vi "Dashboard Main.vi"() -> ()   [LabVIEW 2018]
uses:
  <vilib>/Utility/miscctls.llb/LVRowAndColumnTypeDef.ctl
  <vilib>/event_ctls.llb/eventvkey.ctl
  <vilib>/Rock Robotics/Network Tables/NT Read Numeric Array.vi
  <vilib>/Rock Robotics/Network Tables/NT Write Boolean.vi
  <vilib>/Rock Robotics/WPI/Dashboard/WPI_DashboardLogging Global.vi
  <vilib>/Rock Robotics/Network Tables/NT Write Numeric Array.vi
  <vilib>/Rock Robotics/Network Tables/NT Read Boolean Array.vi
panel:
  out "Time":dbl
  out "Boolean Array":bool[](array[boolean])
  in  "Key Binds":u16[](array[ring]) items=["No Function", "Gear Shift", "Direction Toggle", "Cube Up", "Cube Down", "LRamp Deploy", "RRamp Deploy", "LRamp Raise", "RRamp Raise"]
  in  "Turning Multiplier":dbl=1.0 format="%#_13g"
  in  "Control System":T1(ring)
  out "error out 2":errorcluster
  out "Profile Name":string="Profile1"
  in  "Load":bool
  in  "Save":bool
  in  "High Gear Turning Multiplier":dbl=0.65 format="%#_13g"
  in  "Turning Deadzone":dbl=0.4 format="%#_13g"
  in  "Foreward Deadzone":dbl=1.0 format="%#_13g"
  in  "Max Speed":dbl=1.0 format="%#_13g"
  in  "Autoshift":bool=TRUE
  in  "Direction Toggle":bool=TRUE
  in  "High Gear":bool=TRUE
  in  "Camera Settings Right":T2={"Frame Rate"=30, "Compression"=30, "Size"=1, "DB Camera Config"=FALSE} {"Frame Rate" scale=1.0..30.0; "Compression" scale=100.0..-1.0; "Size" items=["640x480", "320x240", "160x120"]}
  in  "Camera Name Right":string(combo)="No Camera Selection"
  out "Camera Perf":string
  in  "Camera Settings":T2={"Frame Rate"=30, "Compression"=30, "Size"=1, "DB Camera Config"=FALSE} {"Frame Rate" scale=1.0..30.0; "Compression" scale=100.0..-1.0; "Size" items=["640x480", "320x240", "160x120"]}
  in  "TCP":refnum<k5>
  in  "Rec Mode":enum32{"Stop", "Record", "Playback"}(radio)
  out "Robot IP":string
  out "Image Message":string="Timeout in Camera Communications"
  in  "Dashboard Tab":T3(tab)
  in  "Select Auto":string(combo)="Select Autonomous ..."
  out "NT Connection":bool
  out "MotorChart R":cluster{"Numeric":dbl, "Numeric":dbl}(graph)
  out "MotorChart L":cluster{"Numeric":dbl, "Numeric":dbl}(graph)
  out "MotorSliders R":cluster{"MotorSlide1":dbl, "MotorSlide2":dbl} {"MotorSlide2" scale=-1.0..1.0 scale format="%#_2e"; "MotorSlide1" scale=-1.0..1.0 scale format="%#_2e"}
  out "MotorSliders L":cluster{"MotorSlide1":dbl, "MotorSlide2":dbl} {"MotorSlide2" scale=-1.0..1.0 scale format="%#_2e"; "MotorSlide1" scale=-1.0..1.0 scale format="%#_2e"}
  out "Gyro":dbl(knob) scale=0.0..360.0
  out "JS1 Z":dbl(slide) scale=-1.0..1.0 scale format="%#_2e"
  out "JS1 Graph":cluster{"X":dbl, "Y":dbl}[](graph)
  out "JS1 Buttons":T4
  out "JS2 Z":dbl(slide) scale=-1.0..1.0 scale format="%#_2e"
  out "JS2 Graph":cluster{"X":dbl, "Y":dbl}[](graph)
  out "JS2 Buttons":T4
  out "Mode":T5(ring)=enum."Auto Disabled"
  out "Right Camera Perf":cluster{"Bandwidth (Mbps)":dbl, "FPS":dbl}
  out "Camera Image Right":T6(plugin-control)
  in  "DB/String 9":string
  in  "DB/String 8":string
  in  "DB/String 7":string
  in  "DB/String 6":string
  in  "DB/String 5":string
  in  "DB/String 4":string
  in  "DB/String 3":string
  in  "DB/String 2":string
  in  "DB/String 1":string
  in  "DB/String 0":string
  in  "DB/Slider 0":dbl(slide) scale=0.0..5.0
  in  "DB/Slider 1":dbl(slide) scale=0.0..5.0
  in  "DB/Slider 2":dbl(slide) scale=0.0..5.0
  in  "DB/Slider 3":dbl(slide) scale=0.0..5.0
  out "DB/LED 3":bool
  out "DB/LED 2":bool
  out "DB/LED 1":bool
  out "DB/LED 0":bool
  in  "DB/Button 3":bool
  in  "DB/Button 2":bool
  in  "DB/Button 1":bool
  in  "DB/Button 0":bool caption="New Name"
  in  "Toggle Interpolation":bool
  out "XY Graph":cluster{dbl[], dbl[]}(graph)
  in  "Add Cursor":bool
  in  "Interpolation Method":i32(ring)=1 items=["nearest", "linear", "spline", "cubic Hermite", "Lagrange"]
  in  "Graph Points":i32
  in  "Remove Cursor":bool
  in  "Test Slider":dbl(slide) scale=0.0..100.0 scale format="%#_3g"
  in  "On/Off":bool caption="Solenoid"
  in  "Test Name":u16(ring) items=["Select the test to run..."]
  in  "Test Tree":string(tree)
  in  "Motor":cluster{"Value":dbl, "Enable":bool} {"Value" scale=-1.0..1.0 scale format="%#_3g"}
  out "Progress":T7 {"Test Progress" scale=0.0..100.0}
  in  "Rev/Fwd":cluster{"Forward":bool, "Reverse":bool}
  in  "Test Ring":u16(ring) items=["Monochrome", "Color"]
  out "Cmd Status":string
  in  "Execute Command":bool
  in  "Command Params":string[][](table)
  in  "Command Selection":i32(listbox)
  in  "CheckList":i32(listbox)
  out "Tree":string(tree)
  out "Camera Image":T6(plugin-control)
  out "Background":bool
  in  "Camera Name":string(combo)="No Camera Selection"
  # "HW"
  # "HW"
  # "Raw Joystick"
  # "Interpolated Joystick"
  # "Drive Motors"
  # "Front"
  # "Right"
  # "Left"
  # "Back"
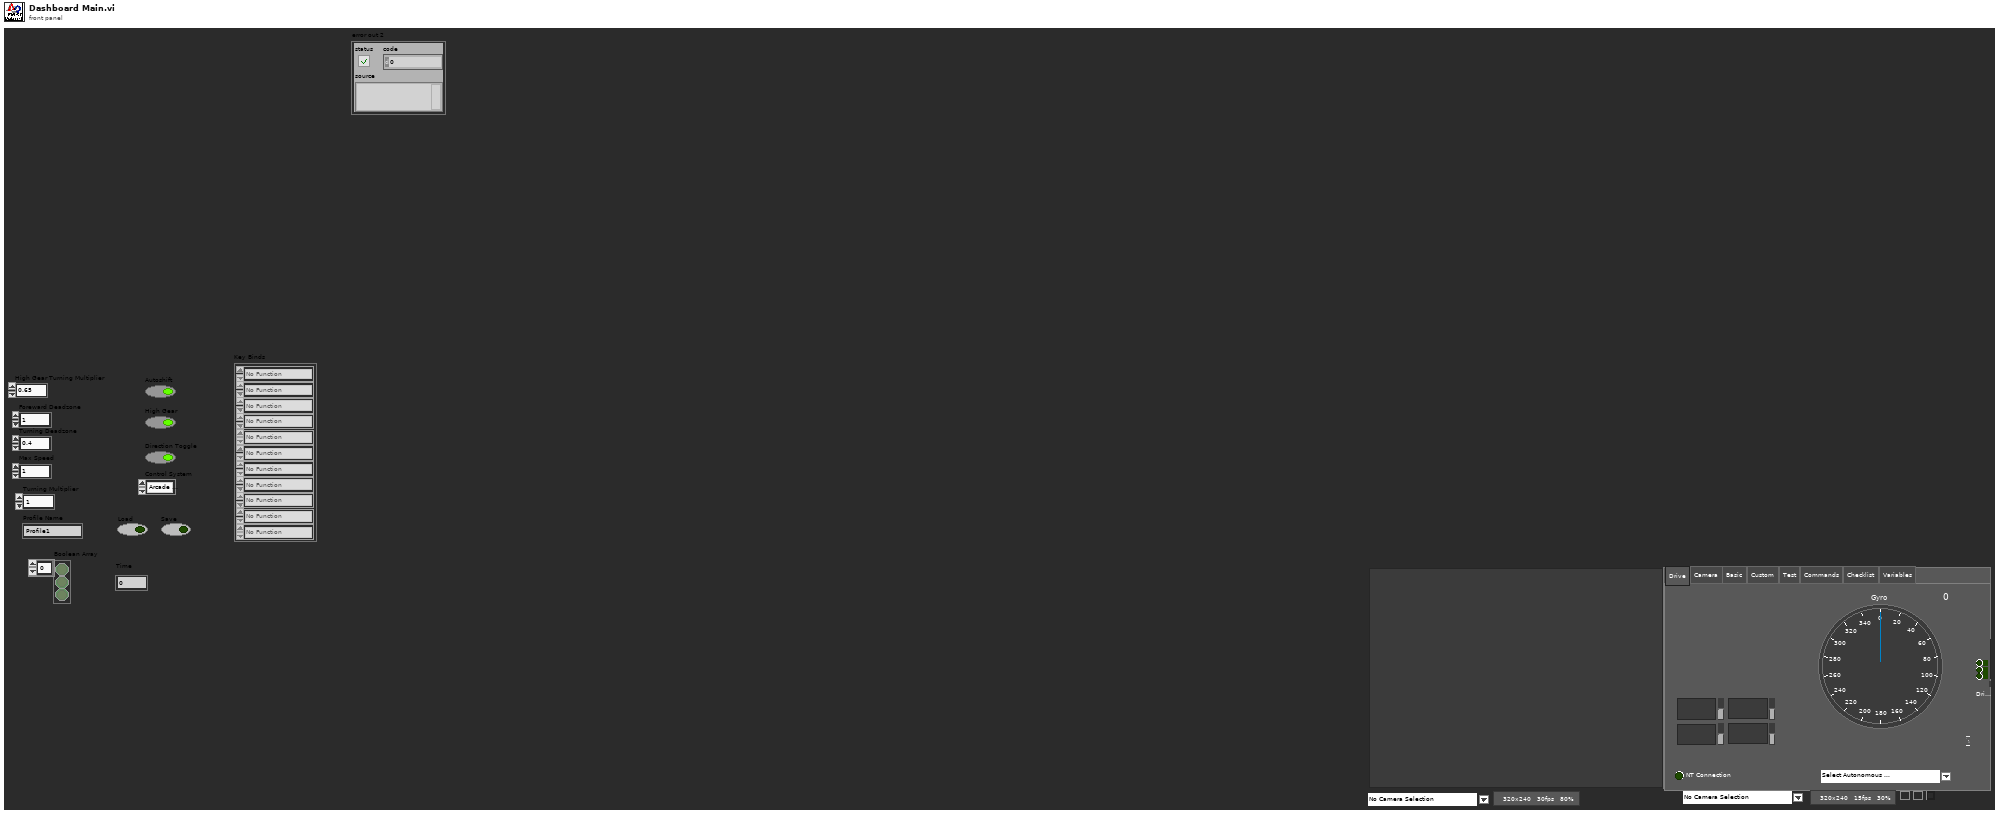
[diagram p1: front panel]
types:
  T1 = enum16{"Arcade Drive", "Two Part Arcade Drive", "Tank"}
  T2 = cluster{"Frame Rate":i32, "Compression":i32, "Size":u16, "DB Camera Config":bool}
  T3 = enum32{"Drive", "Camera", "Basic", "Custom", "Test", "Commands", "Checklist", "Variables"}
  T4 = cluster{bool, bool, bool, bool, bool, bool, bool, bool, bool, bool, bool, bool}
  T5 = enum8{"Tele-Op Disabled", "Tele-Op Enabled", "Auto Disabled", "Auto Enabled", "Test Disabled", "Test Enabled", "Disconnected", "No Code", "E-Stop"}
  T6 = typedef "IMAQ Image.ctl" = refnum<image>
  T7 = cluster{"Test Progress":u8, "Test Progress Text":string}
  T8 = cluster{"Save Path":path, "Interval (s)":dbl, "Keep":i32}
  T9 = typedef "Image Type" = u32
  T10 = cluster{"IDs":cluster{"RPC field ID":u16, "Unique ID":u16}, "String":string}
  T11 = cluster{"High Gear Turning Multiplier":refnum<vi>, "Turning Deadzone":refnum<vi>, "Foreward Deadzone":refnum<vi>, "Max Speed":refnum<vi>, "Autoshift":refnum<vi>, "High Gear":refnum<vi>, "Direction Toggle":refnum<vi>, "Control System":refnum<vi>, "Turning Multiplier":refnum<vi>, "Profile Name":refnum<vi>, "Key Binds":refnum<vi>}
  T12 = cluster{"Error Strings":string, "Disable Counts":cluster{u16, u16}, "Rail Faults":cluster{u16, u16, u16}, "Robot IP":string, "DB Mode":u8, "Event Info":cluster{"Name":string, "Type":u8, "Number":u16, "Replay":u8}}
  T13 = cluster{"Storage":cluster{"Disk Free":u64, "RAM Block":u32, "RAM free":u32}, "CPU Utilization":cluster{"CPU % ISR":sgl, "CPU % Time Crit":sgl, "CPU % Timed Str":sgl, "CPU % High":sgl, "CPU % Above":sgl, "CPU % Normal":sgl, "CPU % Low":sgl}, "CAN":cluster{"% Bus Utilization":sgl, "Bus Off Cnt":u32, "TX_FIFO Full Cnt":u32, "Receive Error Cnt":u8, "Transmit Error Cnt":u8}, "HID":cluster{"HID Outputs":u32, "Rumble Low":u16, "Rumble High":u16}[]}
  T14 = cluster{"Status bits":cluster{"Test Mode":bool, "Autonomous":bool, "Enabled":bool, "Code Start":bool, "Brownout":bool, "Reserved 2":bool, "Reserved 3":bool, "E-Stop":bool}, "Code Trace":cluster{"Disabled":bool, "TeleOp":bool, "Auto":bool, "Test":bool}, "Controller Type":enum16{"unknown", "cRIO", "roboRio"}, "Code?":enum16{"unknown", "noCode", "code"}, "Battery V":dbl}
  T15 = cluster{"Control Bits":cluster{"TestMode":bool, "Autonomous":bool, "Enabled":bool, "FMS Present":bool, bool, bool, bool, "E-Stop":bool}, "Team Station ":u8, "Countdown":sgl, "Joystick Values":cluster{"Axes":dbl[], "Buttons":bool[], "POVs":i16[]}[]}
  T16 = cluster{"Axes":dbl[], "Buttons":bool[], "POVs":i16[]}[]
  T17 = cluster{"Axes":dbl[], "Buttons":bool[], "POVs":i16[]}
  T18 = cluster{"Buttons[0]":bool, "Buttons[1]":bool, "Buttons[2]":bool, "Buttons[3]":bool, "Buttons[4]":bool, "Buttons[5]":bool, "Buttons[6]":bool, "Buttons[7]":bool, "Buttons[8]":bool, "Buttons[9]":bool, "Buttons[10]":bool, "Buttons[11]":bool}
  T19 = cluster{"Camera Image":refnum<vi>, "Dashboard Tab":refnum<vi>, "Background":refnum<vi>, "Rec Mode":refnum<vi>, "Test Slider":refnum<vi>, "On/Off ":refnum<vi>, "Test Ring":refnum<vi>, "Rev/Fwd":refnum<vi>, "Test Name":refnum<vi>, "Motor":refnum<vi>, "Progress":refnum<vi>, "CheckList":refnum<vi>, "Tree":refnum<vi>, "Test Tree":refnum<vi>, "Command Params":refnum<vi>, "Command Selection":refnum<vi>, "Execute Command":refnum<vi>, "Cmd Status":refnum<vi>, "Camera Settings":refnum<vi>, "Camera Name":refnum<vi>, "Camera Perf":refnum<vi>, "Camera Settings Right":refnum<vi>, "Camera Name Right":refnum<vi>, "Camera Image Right":refnum<vi>}
  T20 = cluster{"Global Rectangle":i32[], "Contours":cluster{"Contour Type":u32, "ROI Type":u32, "Points":i32[]}[]}
  T21 = cluster{"Camera Name Right":string, string, "Saved DB Images Info":cluster{"Save Path":path, "Interval (s)":dbl, "Keep":i32}}
  T22 = cluster{"Camera Name":string, string, "Saved DB Images Info":cluster{"Save Path":path, "Interval (s)":dbl, "Keep":i32}}
  T23 = cluster{"Operation":enum16{"Update", "Clear"}, "Color Box":u32}[]
  T24 = typedef "eventvkey.ctl" = enum16{"ASCII", "Enter", "Return", "Shift", "Ctrl", "Alt", "Cmd", "Opt", "Caps", "NumLock", "Clear", "Break", "Up", "Down", "Left", "Right", "Insert", "Delete", "Home", "End", "PageUp", "PageDown", "Escape", "Help", "Pause", "ScrollLock", "F1", "F2", "F3", "F4", "F5", "F6", "F7", "F8", "F9", "F10", "F11", "F12", "F13", "F14", "F15", "F16", "F17", "F18", "F19", "F20", "F21", "F22", "F23", "F24", "Play", "VolumeUp", "VolumeDown", "Mute", "Two Byte Char"}
  T25 = cluster{"Image Size":bool, "Image Type":bool, "Pixel Value":bool, "ROI Information":bool, "Zoom Factor":bool}
  T26 = cluster{"Operation":enum16{"Update", "Clear"}, "Color Box":u32}
  T27 = typedef "LVRowAndColumnTypeDef.ctl" = cluster{"Row":i32, "Column":i32}
  T28 = cluster{"Shift":bool, "Ctrl":bool, "Alt":bool, "Cmd":bool, "Opt":bool}
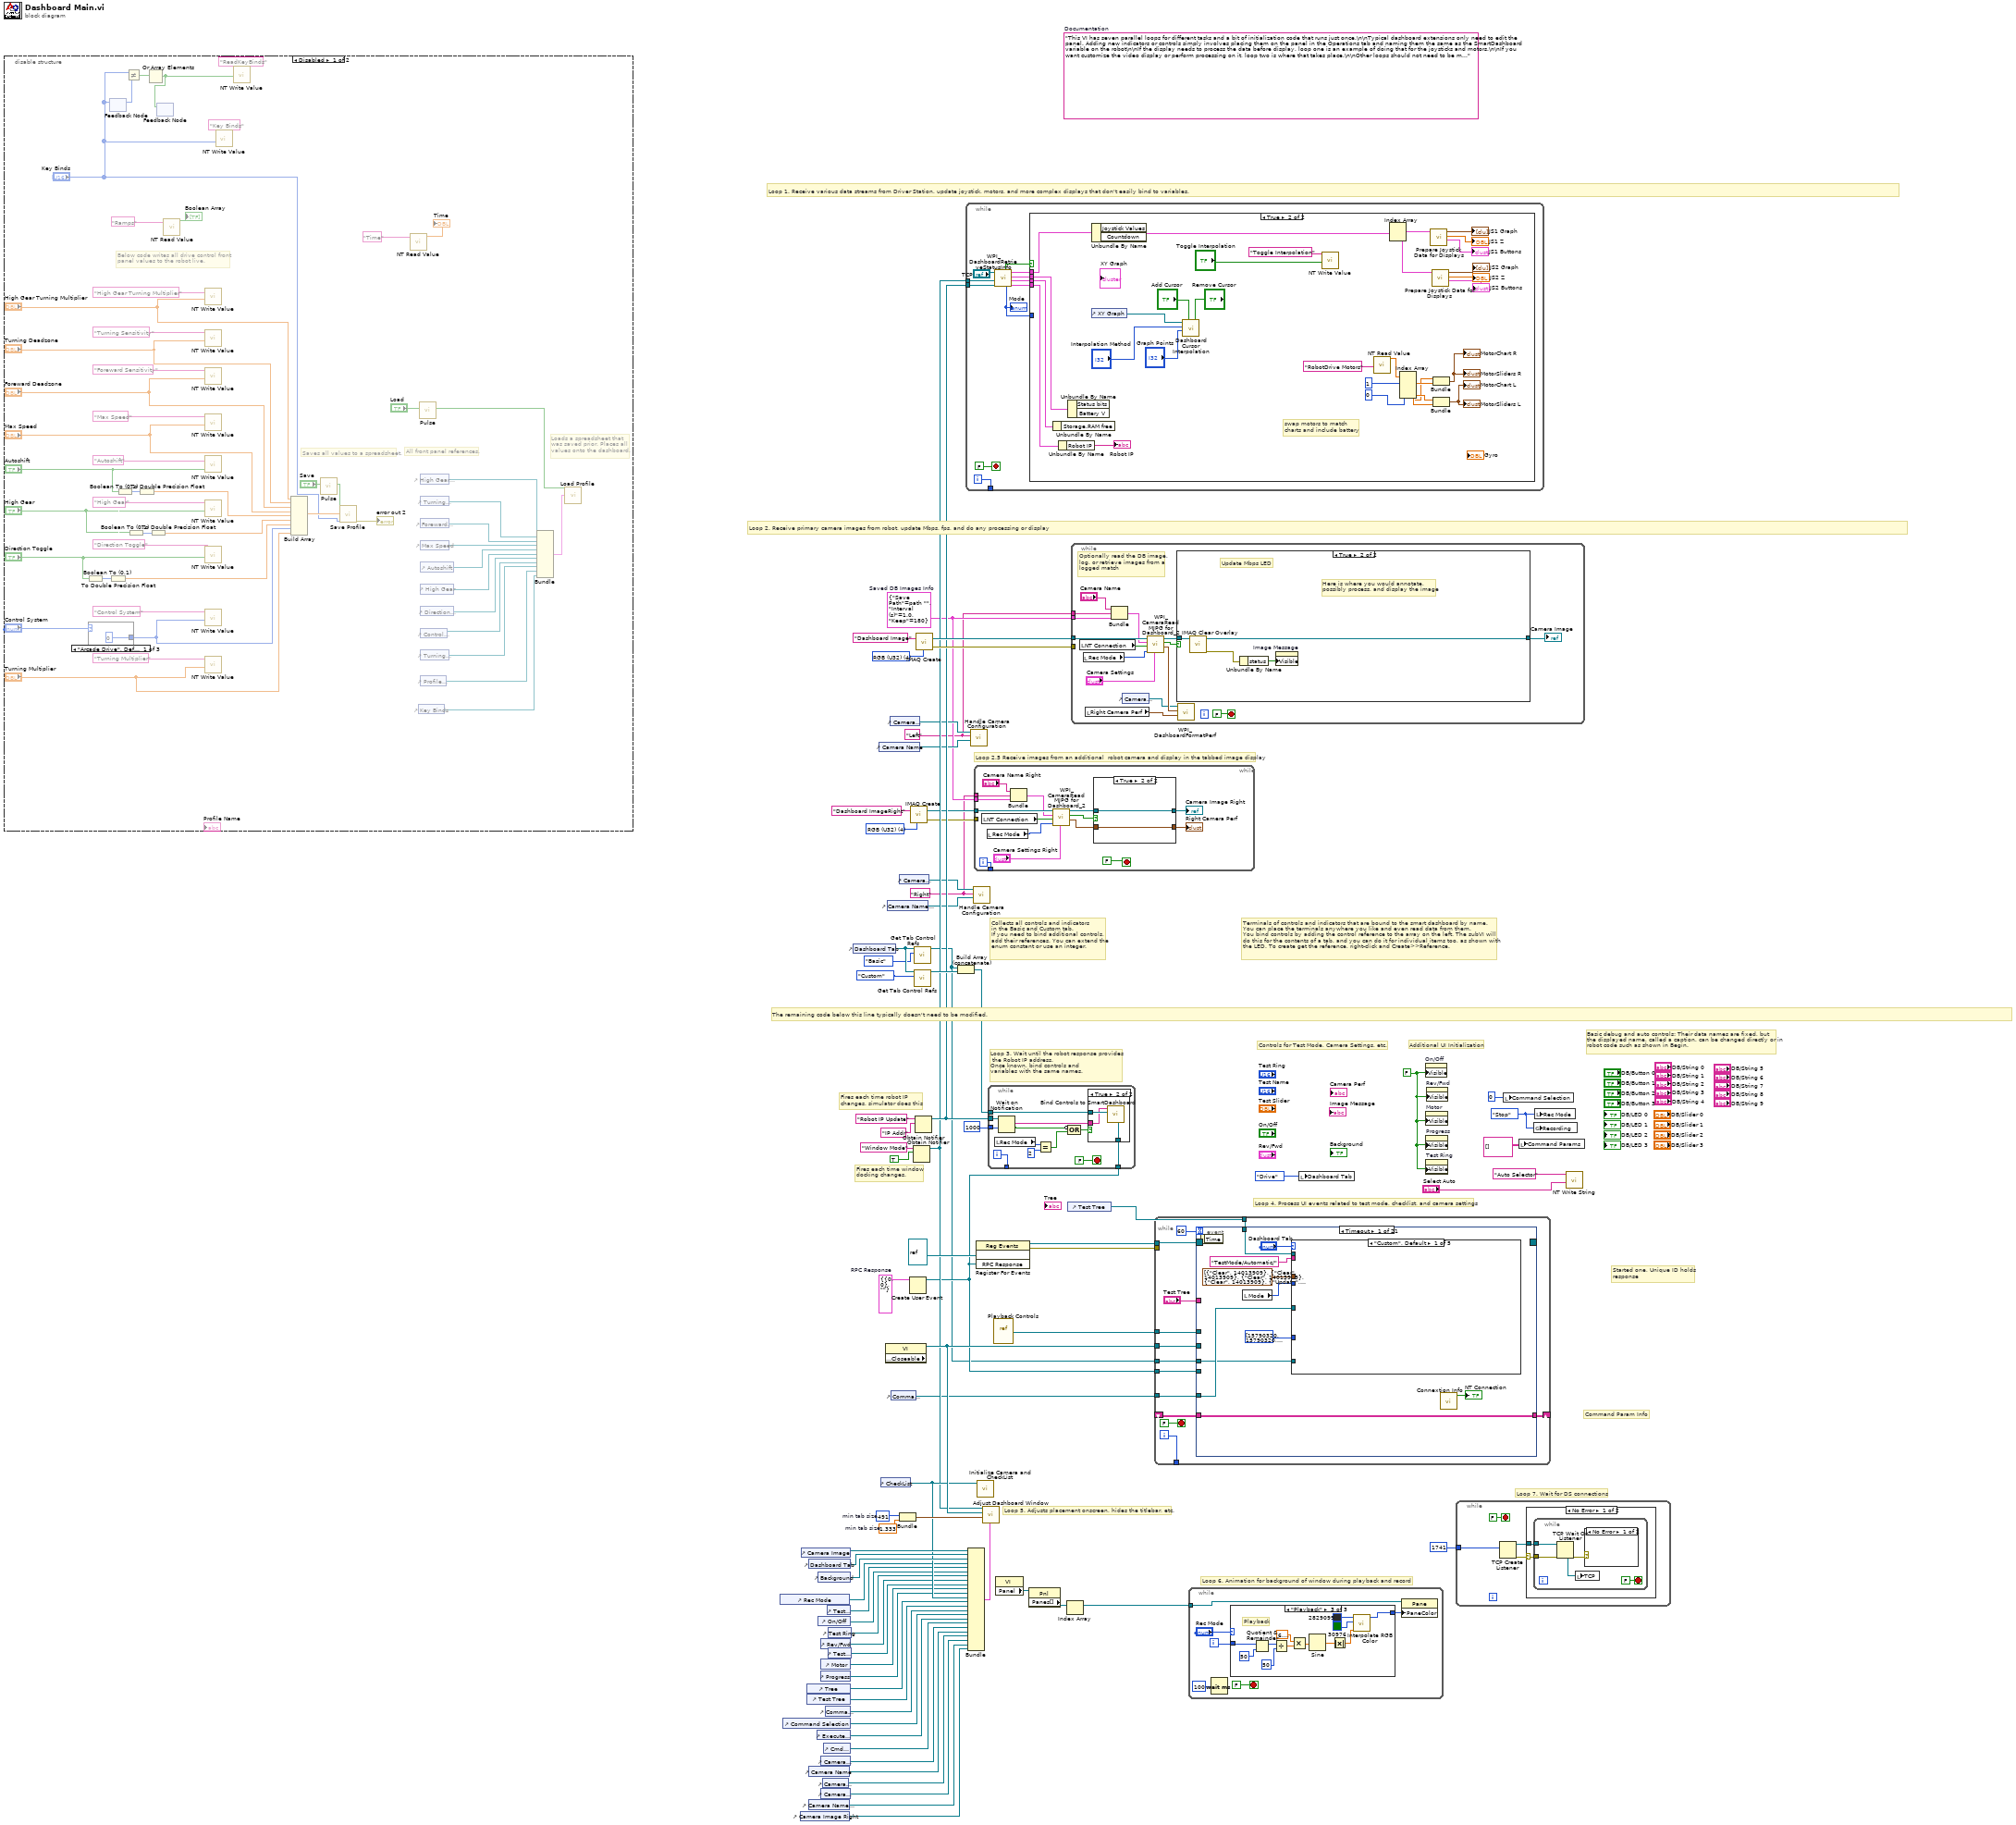
[diagram p0: block diagram]
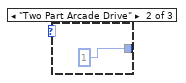
[diagram p2: hidden frame]
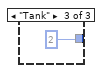
[diagram p3: hidden frame]
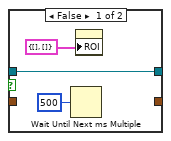
[diagram p5: hidden frame]
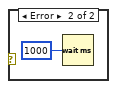
[diagram p6: hidden frame]
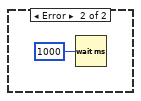
[diagram p7: hidden frame]
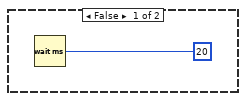
[diagram p8: hidden frame]
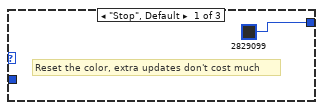
[diagram p9: hidden frame]
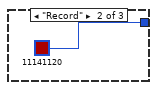
[diagram p10: hidden frame]
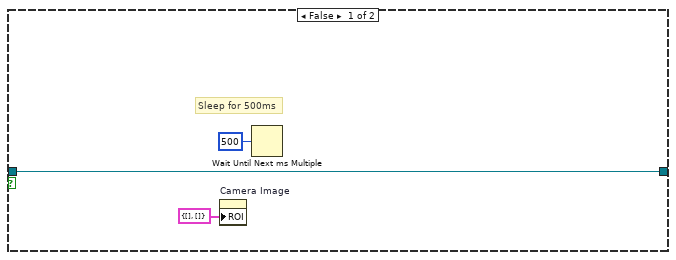
[diagram p12: hidden frame]
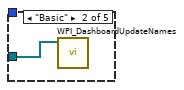
[diagram p13: hidden frame]
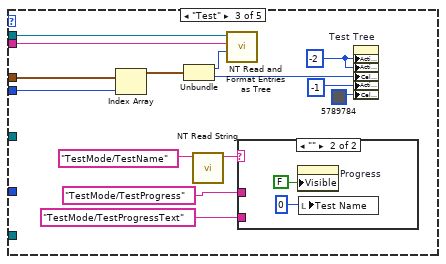
[diagram p14: hidden frame]
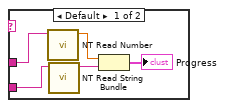
[diagram p15: hidden frame]
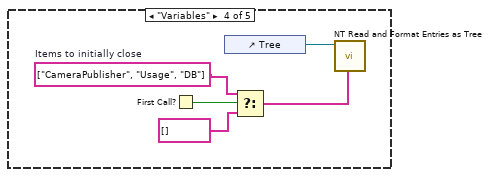
[diagram p16: hidden frame]
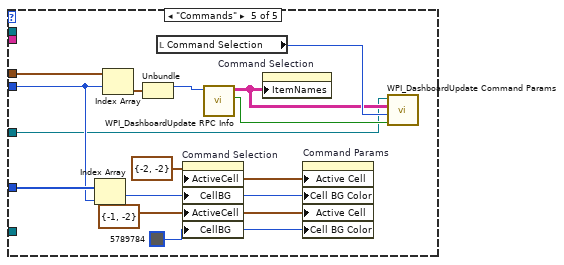
[diagram p17: hidden frame]
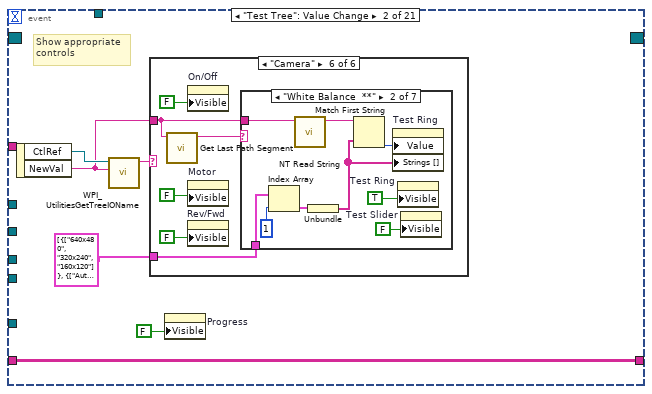
[diagram p18: hidden frame]
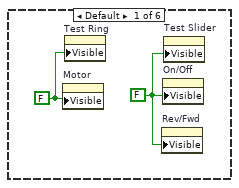
[diagram p19: hidden frame]
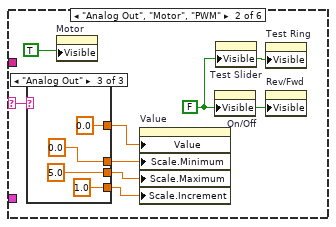
[diagram p20: hidden frame]
diagram:
  w3 = T8 {"Save Path"=path "", "Interval (s)"=1.0, "Keep"=180}  # Saved DB Images Info
  w2 = "Right"
  w1 = "Left"
  w13 = T9 4 items=["Grayscale (U8)", "Grayscale (I16)", "Grayscale (SGL)", "Complex (CSG)", "RGB (U32)", "HSL (U32)", "RGB (U64)"] ("Image Type")
  w29 = T10 {"IDs"={"RPC field ID"=0, "Unique ID"=0}, "String"=""}  # RPC Response
  w52 = 491  # min tab size
  w51 = 1.333  # min tab size
  w59 = enum32{"Stop", "Record", "Playback"}."Stop" ("Rec Mode")
  w36 = FALSE ("Visible")
  (unwired) "This VI has seven parallel loops for different tasks and a bit of initialization code that runs just once.\n\nTypical dashboard extensions only need to edit the panel. Adding new indicators or controls simply involves placing them on the panel in the Operations tab and naming them the same as the SmartDashboard variable on the robot\n\nIf the display needs to process the data before display, loop one is an example of doing that for the joysticks and motors.\n\nIf you want customize the video display or perform processing on it, loop two is where that takes place.\n\nOther loops should not need to be modified. They are pretty standard, and document the task they perform."  # Documentation
  w76 = T9 4 items=["Grayscale (U8)", "Grayscale (I16)", "Grayscale (SGL)", "Complex (CSG)", "RGB (U32)", "HSL (U32)", "RGB (U64)"] ("Image Type")
  # "Loop 2.5 Receive images from an additional  robot camera and display in the tabbed image display"
  # "Command Param Info"
  # "Started one, Unique ID holds\nresponse"
  # "Loop 7. Wait for DS connections"
  # "Basic debug and auto controls: Their data names are fixed, but\nthe displayed name, called a caption, can be changed directly or in\nrobot code such as shown in Begin."
  # "Controls for Test Mode, Camera Settings, etc."
  # "Additional UI Initialization"
  # "Loop 6. Animation for background of window during playback and record"
  # "Fires each time robot IP\nchanges, simulator does this"
  # "Fires each time window\ndocking changes."
  # "Collects all controls and indicators\nin the Basic and Custom tab.\nIf you need to bind additional controls,\nadd their references. You can extend the\nenum constant or use an integer."
  # "The remaining code below this line typically doesn't need to be modified."
  # "Loop 4. Process UI events related to test mode, checklist, and camera settings"
  # "Terminals of controls and indicators that are bound to the smart dashboard by name.\nYou can place the terminals anywhere you like and even read data from them.\nYou bind controls by adding the control reference to the array on the left. The subVI will\ndo this for the contents of a tab, and you can do it for individual items too, as shown with\nthe LED. To create get the reference, right-click and Create>>Reference."
  # "Loop 3. Wait until the robot response provides\n the Robot IP address.\nOnce known, bind controls and\nvariables with the same names."
  # "Loop 5. Adjusts placement onscreen, hides the titlebar, etc."
  # "Loop 1. Receive various data streams from Driver Station, update joystick, motors, and more complex displays that don't easily bind to variables."
  # "Loop 2. Receive primary camera images from robot, update Mbps, fps, and do any processing or display"
  n1 = disable-structure shown="Disabled" {
    frame Disabled {
      # "Loads a spreadsheet that\nwas saved prior. Places all\nvalues onto the dashboard."
      # "All front panel references."
      # "Saves all values to a spreadsheet."
      # "Below code writes all drive control front\npanel values to the robot live."
      n2 = Boolean To (0,1)(Boolean="Direction Toggle") -> (0, 1=w112:i16)
      n3 = case shown="\"Arcade Drive\", Default" "Control System" {
        tunnel: [0 1 2] -> w89
        frame "Arcade Drive", Default {
        }
        frame "Two Part Arcade Drive" {
        }
        frame "Tank" {
        }
      }
      n4 = feedback #1() -> (w88:u16[])  [unwired: 1 in]
      n5 = feedback-in #1("Key Binds") -> ()
      n6 = To Double Precision Float(number=w112) -> (double precision float=w113:dbl)
      n7 = Boolean To (0,1)(Boolean="Autoshift") -> (0, 1=w108:i16)
      n8 = Not Equal?(x="Key Binds", y=w88) -> (x != y?=w87:bool[])
      n9 = Boolean To (0,1)(Boolean="High Gear") -> (0, 1=w110:i16)
      n10 = To Double Precision Float(number=w108) -> (double precision float=w109:dbl)
      n11 = Or Array Elements(Boolean array=w87) -> (logical OR=w85:bool)
      n12 = To Double Precision Float(number=w110) -> (double precision float=w111:dbl)
      n13 = feedback #2() -> ()  [unwired: 2 in]
      n14 = feedback-in #2(w85) -> ()
      n15 = call-poly <vilib>:"NT Read Value.vi"("Name"="Ramps") -> ("Boolean Array"=→"Boolean Array":bool[])  [unwired: 9 in, 1 out]
      n16 = call-poly <vilib>:"NT Write Value.vi"("Numeric"="High Gear Turning Multiplier", "Name"="High Gear Turning Multiplier") -> ()  [unwired: 9 in, 1 out]
      n17 = call-poly <vilib>:"NT Write Value.vi"("Numeric"="Turning Deadzone", "Name"="Turning Sensitivity") -> ()  [unwired: 9 in, 1 out]
      n18 = call-poly <vilib>:"NT Write Value.vi"("Numeric"="Foreward Deadzone", "Name"="Foreward Sensitivity") -> ()  [unwired: 9 in, 1 out]
      n19 = call-poly <vilib>:"NT Write Value.vi"("Numeric"="Max Speed", "Name"="Max Speed") -> ()  [unwired: 9 in, 1 out]
      n20 = call-poly <vilib>:"NT Write Value.vi"("Boolean"="Autoshift", "Name"="Autoshift") -> ()  [unwired: 9 in, 1 out]
      n21 = call-poly <vilib>:"NT Write Value.vi"("Boolean"="High Gear", "Name"="High Gear") -> ()  [unwired: 9 in, 1 out]
      n22 = call-poly <vilib>:"NT Write Value.vi"("Boolean"="Direction Toggle", "Name"="Direction Toggle") -> ()  [unwired: 9 in, 1 out]
      n23 = call-poly <vilib>:"NT Write Value.vi"("Numeric"=w89, "Name"="Control System") -> ()  [unwired: 9 in, 1 out]
      n24 = call-poly <vilib>:"NT Write Value.vi"("Numeric"="Turning Multiplier", "Name"="Turning Multiplier") -> ()  [unwired: 9 in, 1 out]
      n25 = call-poly <vilib>:"NT Write Value.vi"("Numeric Array"="Key Binds", "Name"="Key Binds") -> ()  [unwired: 9 in, 1 out]
      n26 = call-poly <vilib>:"NT Write Value.vi"("Boolean"=w85, "Name"="ReadKeyBinds") -> ()  [unwired: 9 in, 1 out]
      n27 = Build Array("High Gear Turning Multiplier", "Turning Deadzone", "Foreward Deadzone", "Max Speed", w109, w111, w113, w89, "Turning Multiplier") -> (w115:dbl[])
      n28 = call "Pulse.vi"("Input"="Save") -> ("Output"=w107:bool)  [unwired: 10 in]
      n29 = call "Save Profile.vi"("Key Binds"="Key Binds", "Driver Pref"=w115, "Output"=w107) -> ("error out"=→"error out 2":errorcluster)  [unwired: 8 in]
      n30 = call-poly <vilib>:"NT Read Value.vi"("Name"="Time") -> ("Numeric"=→"Time":dbl)  [unwired: 9 in, 1 out]
      n31 = control-ref of="Key Binds"() -> (w83:refnum<vi>)
      n32 = call "Pulse.vi"("Input"="Load") -> ("Output"=w104:bool)  [unwired: 10 in]
      n33 = control-ref of="Profile Name"() -> (w92:refnum<vi>)
      n34 = control-ref of="High Gear Turning Multiplier"() -> (w103:refnum<vi>)
      n35 = control-ref of="Turning Deadzone"() -> (w102:refnum<vi>)
      n36 = control-ref of="Foreward Deadzone"() -> (w101:refnum<vi>)
      n37 = control-ref of="Max Speed"() -> (w100:refnum<vi>)
      n38 = control-ref of="Autoshift"() -> (w99:refnum<vi>)
      n39 = control-ref of="High Gear"() -> (w98:refnum<vi>)
      n40 = control-ref of="Direction Toggle"() -> (w97:refnum<vi>)
      n41 = control-ref of="Control System"() -> (w95:refnum<vi>)
      n42 = control-ref of="Turning Multiplier"() -> (w91:refnum<vi>)
      n43 = Bundle("High Gear Turning Multiplier"=w103, "Turning Deadzone"=w102, "Foreward Deadzone"=w101, "Max Speed"=w100, "Autoshift"=w99, "High Gear"=w98, "Direction Toggle"=w97, "Control System"=w95, "Turning Multiplier"=w91, "Profile Name"=w92, "Key Binds"=w83) -> (w82:T11)  [unwired: 1 in]
      n44 = call "Load Profile.vi"("Output"=w104, "References"=w82) -> ()  [unwired: 14 in]
    }
    frame Enabled {
    }
  }
  n45 = control-ref of="Rec Mode"() -> (w42:refnum<vi>)
  n46 = control-ref of="Command Selection"() -> (w28:refnum<vi>)
  n47 = control-ref of="Camera Image Right"() -> (w6:refnum<vi>)
  n48 = control-ref of="Camera Image"() -> (w54:refnum<vi>)
  n49 = control-ref of="Tree"() -> (w46:refnum<vi>)
  n50 = control-ref of="Test Tree"() -> (w45:refnum<vi>)
  n51 = control-ref of="Dashboard Tab"() -> (w53:refnum<vi>)
  n52 = control-ref of="Camera Name"() -> (w19:refnum<vi>)
  n53 = control-ref of="Camera Name Right"() -> (w7:refnum<vi>)
  n54 = control-ref of="Execute Command"() -> (w30:refnum<vi>)
  n55 = control-ref of="Background"() -> (w49:refnum<vi>)
  n56 = control-ref of="On/Off"() -> (w40:refnum<vi>)
  n57 = control-ref of="Progress"() -> (w37:refnum<vi>)
  n58 = control-ref of="Camera Settings"() -> (w20:refnum<vi>)
  n59 = control-ref of="Camera Settings Right"() -> (w8:refnum<vi>)
  n60 = control-ref of="Rev/Fwd"() -> (w38:refnum<vi>)
  n61 = control-ref of="Motor"() -> (w43:refnum<vi>)
  n62 = control-ref of="Camera Perf"() -> (w18:refnum<vi>)
  n63 = control-ref of="Cmd Status"() -> (w24:refnum<vi>)
  n64 = control-ref of="Command Params"() -> (w31:refnum<vi>)
  n65 = control-ref of="Test Slider"() -> (w41:refnum<vi>)
  n66 = control-ref of="Test Ring"() -> (w39:refnum<vi>)
  n67 = control-ref of="Test Name"() -> (w44:refnum<vi>)
  n68 = control-ref of="Dashboard Tab"() -> (w57:refnum<vi>)
  n69 = control-ref of="Camera Name"() -> (w21:refnum<vi>)
  n70 = control-ref of="CheckList"() -> (w47:refnum<vi>)
  n71 = property class="VI" props=["Front Panel.Closeable"]() -> (reference out=w58:refnum<vi>)  [unwired: 2 in, 2 out]
  n72 = control-ref of="Camera Name Right"() -> (w9:refnum<vi>)
  n73 = control-ref of="Camera Settings"() -> (w22:refnum<vi>)
  n74 = control-ref of="Command Params"() -> (w23:refnum<vi>)
  n75 = control-ref of="Camera Settings Right"() -> (w10:refnum<vi>)
  n76 = Bundle("min tab size"=w52, "min tab size"=w51) -> (w50:cluster{"min tab size":i32, "min tab size":dbl})  [unwired: 1 in]
  n77 = Create User Event(user event datatype=w29) -> (user event=w25:refnum<user-event>)  [unwired: 1 in, 1 out]
  n78 = call "IMAQ Create"("Image Name"="Dashboard ImageRight", "Image Type"=w13) -> ("New Image"=w12:T6, "error out"=w11:errorcluster)  [unwired: 2 in, 1 out]
  n79 = Obtain Notifier(name (unnamed)="Window Mode", notification data type=TRUE) -> (notifier out=w34:refnum<notifier>)  [unwired: 2 in, 2 out]
  n80 = call <vilib>:"Get Tab Control Refs.vi"("Page Index"=T3."Basic" ("Dashboard Tab"), "TabControl in"=w57) -> ("ControlsOnPage"=w17:refnum<vi>[])  [unwired: 9 in]
  n81 = call <vilib>:"Get Tab Control Refs.vi"("Page Index"=T3."Custom" ("Dashboard Tab"), "TabControl in"=w57) -> ("ControlsOnPage"=w56:refnum<vi>[])  [unwired: 9 in]
  n82 = Obtain Notifier(name (unnamed)="Robot IP Update", notification data type="IP Addr" ("name (unnamed)")) -> (notifier out=w35:refnum<notifier>)  [unwired: 2 in, 2 out]
  n83 = call "IMAQ Create"("Image Name"="Dashboard Image", "Image Type"=w76) -> ("New Image"=w74:T6, "error out"=w73:errorcluster)  [unwired: 2 in, 1 out]
  n84 = Build Array (concatenate)(w17, w56) -> (w55:refnum<vi>[])
  n85 = while {
    tunnel: [w142] -> _
    tunnel: w35 -> [w136]
    tunnel: w34 -> [w133]
    i -> [w142]
    stop <- FALSE stop-if-true
    n86 = call <vilib>:"WPI_DashboardRetrieveStatusInfo.vi"("Binding Refnum"=w136, "Window Mode Notifier"=w133, "TCP Cnx"="TCP") -> ("Power and Errors"=w137:T12, "Robot Metrics"=w140:T13, "Status Info"=w141:T14, "Control Info"=w138:T15, "Robot Mode"=w135:T5, "Process?"=w139:bool)  [unwired: 3 in]
    "Mode" <- w135
    n87 = case shown="True" w139 {
      tunnel: w141 -> [_ w175]
      tunnel: w140 -> [_ w174]
      tunnel: w138 -> [_ w173]
      tunnel: w137 -> [_ w172]
      tunnel: w135 -> [_ _]
      frame False {
        n88 = Wait (ms)(milliseconds to wait=u32 20) -> ()  [unwired: 1 out]
      }
      frame True {
        # "swap motors to match\ncharts and include battery"
        n89 = Unbundle By Name(w174) -> ()  [unwired: 1 out]
        n90 = Unbundle By Name(w172) -> ("Robot IP"=→"Robot IP":string)
        n91 = Unbundle By Name(w175) -> ()  [unwired: 2 out]
        n92 = control-ref of="XY Graph"() -> (w149:refnum<vi>)
        n93 = Unbundle By Name(w173) -> ("Joystick Values"=w156:T16)  [unwired: 1 out]
        n94 = call "Dashboard Cursor Interpolation.vi"("Remove Cursor"="Remove Cursor", "Add Cursor"="Add Cursor", "Graph Detail"="Graph Points", "Interpolation Method"="Interpolation Method", "Interpolation Points"=w149) -> ()  [unwired: 7 in]
        n95 = call-poly <vilib>:"NT Write Value.vi"("Boolean"="Toggle Interpolation", "Name"="Toggle Interpolation") -> ()  [unwired: 9 in, 1 out]
        n96 = call-poly <vilib>:"NT Read Value.vi"("Name"="RobotDrive Motors") -> ("Numeric Array"=w158:dbl[])  [unwired: 9 in, 1 out]
        n97 = Index Array(array=w156) -> (element #1=w163:T17, element #2=w145:T17)  [unwired: 2 in]
        n98 = Index Array(array=w158, index #1=1, index #4=0) -> (element #1=w167:dbl, element #2=w168:dbl, element #3=w166:dbl, element #4=w171:dbl)  [unwired: 2 in]
        n99 = call "Prepare Joystick Data for Displays.vi"("Joystick Values"=w163) -> ("Buttons"=→"JS1 Buttons":T18, "Z Axis"=→"JS1 Z":dbl, "Cartesian Data"=→"JS1 Graph":cluster{"X axis":dbl, "X axis":dbl}[])  [unwired: 8 in]
        n100 = call "Prepare Joystick Data for Displays.vi"("Joystick Values"=w145) -> ("Buttons"=→"JS2 Buttons":T18, "Z Axis"=→"JS2 Z":dbl, "Cartesian Data"=→"JS2 Graph":cluster{"X axis":dbl, "X axis":dbl}[])  [unwired: 8 in]
        n101 = Bundle("Numeric"=w166, "Numeric"=w167) -> (→"MotorChart R" →"MotorSliders R":cluster{"Numeric":dbl, "Numeric":dbl})  [unwired: 1 in]
        n102 = Bundle("Numeric"=w168, "Numeric"=w171) -> (→"MotorChart L" →"MotorSliders L":cluster{"Numeric":dbl, "Numeric":dbl})  [unwired: 1 in]
      }
    }
  }
  n103 = Bundle("Camera Image"=w54, "Dashboard Tab"=w53, "Background"=w49, "Rec Mode"=w42, "Test Slider"=w41, "On/Off"=w40, "Test Ring"=w39, "Rev/Fwd"=w38, "Test Name"=w44, "Motor"=w43, "Progress"=w37, "CheckList"=w47, "Tree"=w46, "Test Tree"=w45, "Command Params"=w31, "Command Selection"=w28, "Execute Command"=w30, "Cmd Status"=w24, "Camera Settings"=w20, "Camera Name"=w19, "Camera Perf"=w18, "Camera Settings Right"=w8, "Camera Name Right"=w7, "Camera Image Right"=w6) -> (w48:T19)  [unwired: 1 in]
  n104 = call "Handle Camera Configuration.vi"("CameraNameRef"=w21, "Display Name"=w1, "ClusterRef"=w22) -> ()  [unwired: 9 in]
  n105 = call "Handle Camera Configuration.vi"("CameraNameRef"=w9, "Display Name"=w2, "ClusterRef"=w10) -> ()  [unwired: 9 in]
  n106 = while {
    tunnel: w12 -> [w190]
    tunnel: w11 -> [_]
    tunnel: [w185] -> _
    tunnel: w3 -> [w181]
    tunnel: w2 -> [w178]
    i -> [w185]
    stop <- FALSE stop-if-true
    n107 = local read "NT Connection"() -> (w182:bool)
    n108 = local read "Rec Mode"() -> (w189:enum32{"Stop", "Record", "Playback"})
    n109 = Bundle("Camera Name Right"="Camera Name Right", w178, "Saved DB Images Info"=w181) -> (w180:T21)  [unwired: 1 in]
    n110 = call <vilib>:"WPI_CameraRead MJPG for Dashboard_2.vi"("Camera Settings"="Camera Settings Right", "Rec Mode"=w189, "NT Connection"=w182, "Capture Info"=w180, "Image in"=w190) -> ("perf info"=w176:cluster{"Bandwidth (Mbps)":dbl, "fps":dbl}, "Active"=w184:bool, "Image\\ out"=w187:T6)  [unwired: 4 in]
    n111 = case shown="True" w184 {
      tunnel: w187 -> [w192 w195]
      tunnel: [w192 w195] -> w183
      tunnel: [_ w194] -> w177
      tunnel: w176 -> [_ w194]
      frame False {
        n112 = Wait Until Next ms Multiple(millisecond multiple=u32 500) -> ()  [unwired: 1 out]
        n113 = property on="Camera Image Right" class="ImageControl"("ROI"=T20 {"Global Rectangle"=[], "Contours"=[]}) -> ()  [unwired: 2 in, 2 out]
      }
      frame True {
      }
    }
    "Camera Image Right" <- w183
    "Right Camera Perf" <- w177
  }
  n114 = register-events(refnum<vi> refnum, w25) -> (reference out=w63:refnum<event-registration>, error out=w62:errorcluster)  [unwired: 2 in]
  n115 = call "Initialize Camera and CheckList.vi"("ListBox in"=w47) -> ()  [unwired: 11 in]
  n116 = call "Adjust Dashboard Window.vi"("Sizing Refnums"=w48, "Size Constraints"=w50, "VI"=w58, "WIn Mode"=w34) -> ()  [unwired: 8 in]
  n117 = while {
    tunnel: w55 -> [w207]
    tunnel: w35 -> [w205]
    tunnel: [w203] -> _
    tunnel: u32 1000 ("milliseconds to wait") -> [w202]
    tunnel: w25 -> [w196]
    i -> [w203]
    stop <- FALSE stop-if-true
    n118 = local read "Rec Mode"() -> (w198:enum32{"Stop", "Record", "Playback"})
    n119 = Wait on Notification(notifier=w205, timeout in ms (-1)=w202) -> (notification=w204:string, timed out?=w200:bool)  [unwired: 2 in, 2 out]
    n120 = Equal?(x=w198, y=u16 2 ("Rec Mode")) -> (x = y?=w199:bool)
    n121 = Compound Arithmetic op=OR(invert w200, w199) -> (w201:bool)
    n122 = case shown="True" w201 {
      tunnel: w207 -> [_ w210]
      tunnel: w204 -> [_ w209]
      tunnel: w196 -> [_ w208]
      frame False {
      }
      frame True {
        n123 = call <vilib>:"Bind Controls to SmartDashboard.vi"("RPC ref"=w208, "Bound Control Refs"=w210, "Server IP Address"=w209) -> ()  [unwired: 9 in]
      }
    }
  }
  n124 = vi-ref "Playback Controls.vi"() -> (w64:refnum<vi>)
  n125 = property class="VI"() -> ("Panel"=w66:refnum<vi>)  [unwired: 2 in, 2 out]
  n126 = property class="Pnl"(reference=w66) -> ("Panes[]"=w67:refnum<vi>[])  [unwired: 1 in, 2 out]
  n127 = Index Array(array=w67) -> (element=w65:refnum<vi>)  [unwired: 1 in]
  n128 = control-ref of="Test Tree"() -> (w68:refnum<vi>)
  n129 = while {
    tunnel: w74 -> [w224]
    tunnel: w73 -> [_]
    tunnel: w3 -> [w217]
    tunnel: w1 -> [w214]
    stop <- FALSE stop-if-true
    # "Optionally read the DB image,\nlog, or retrieve images from a\nlogged match"
    n130 = local read "NT Connection"() -> (w218:bool)
    n131 = local read "Rec Mode"() -> (w221:enum32{"Stop", "Record", "Playback"})
    n132 = local read "Right Camera Perf"() -> (w212:cluster{"Bandwidth (Mbps)":dbl, "FPS":dbl})
    n133 = Bundle("Camera Name"="Camera Name", w214, "Saved DB Images Info"=w217) -> (w216:T22)  [unwired: 1 in]
    n134 = control-ref of="Camera Perf"() -> (w211:refnum<vi>)
    n135 = call <vilib>:"WPI_CameraRead MJPG for Dashboard_2.vi"("Camera Settings"="Camera Settings", "Rec Mode"=w221, "NT Connection"=w218, "Capture Info"=w216, "Image in"=w224) -> ("perf info"=w213:cluster{"Bandwidth (Mbps)":dbl, "fps":dbl}, "Active"=w222:bool, "Image\\ out"=w223:T6)  [unwired: 4 in]
    n136 = case shown="True" w222 {
      tunnel: w223 -> [w227 w230]
      tunnel: [w227 w229] -> w219
      frame False {
        # "Sleep for 500ms"
        n137 = property on="Camera Image" class="ImageControl"("ROI"=T20 {"Global Rectangle"=[], "Contours"=[]}) -> ()  [unwired: 2 in, 2 out]
        n138 = Wait Until Next ms Multiple(millisecond multiple=u32 500) -> ()  [unwired: 1 out]
      }
      frame True {
        # "Here is where you would annotate,\npossibly process, and display the image"
        # "Update Mbps LED"
        n139 = call "IMAQ Clear Overlay"("Image"=w230) -> ("error out"=w231:errorcluster, "Image Out"=w229:T6)  [unwired: 2 in, 7 out]
        n140 = Unbundle By Name(w231) -> ("status"=w232:bool)
        n141 = property on="Image Message" class="Str"("Visible"=w232) -> ()  [unwired: 2 in, 2 out]
      }
    }
    "Camera Image" <- w219
    n142 = call <vilib>:"WPI_DashboardFormatPerf.vi"("Right Camera Perf"=w212, "Performance"=w213, "String in"=w211) -> ()  [unwired: 9 in]
  }
  n143 = while {
    tunnel: [w242] -> _
    tunnel: w68 -> [w241]
    tunnel: w64 -> [w240]
    tunnel: w63 -> [w239]
    tunnel: w62 -> [_]
    tunnel: w58 -> [w238]
    tunnel: w25 -> [w237]
    tunnel: w23 -> [w236]
    shift-right: [w235] -> _
    shift-left: _ -> [w234]
    tunnel: w17 -> [w233]
    i -> [w242]
    stop <- FALSE stop-if-true
    n144 = event shown="[0] Timeout" {
      selector: w239 -> [_ _ _ _ _ _ _ _ _ _ _ _ _ _ _ _ _ _ _ _ _]
      dyn-events: [_ _ _ _ _ _ _ _ _ _ _ _ _ _ _ _ w502 _ _ _ _] -> _
      timeout: u32 60 ("milliseconds to wait") -> [_ _ _ _ _ _ _ _ _ _ _ _ _ _ _ _ _ _ _ _ _]
      tunnel: w241 -> [w254 _ _ _ _ _ _ _ _ _ _ _ _ _ _ _ _ _ _ _ _]
      tunnel: "Test Tree" -> [_ _ _ _ _ _ _ _ _ _ _ w469 w477 w479 w483 w491 _ _ _ _ _]
      tunnel: w240 -> [_ _ _ _ _ _ _ _ _ _ _ _ _ _ _ _ w504 _ w522 _ _]
      tunnel: w238 -> [_ _ _ _ _ _ _ _ _ _ _ _ _ _ _ _ w500 _ _ _ _]
      tunnel: w237 -> [_ _ _ _ _ _ _ _ _ _ _ _ _ _ _ _ w498 _ _ _ _]
      tunnel: w236 -> [w249 _ _ _ _ _ w420 _ _ _ _ _ _ _ _ _ _ _ _ _ _]
      tunnel: [w248 w297 w399 w404 w413 w417 w418 w427 w437 w444 w456 w468 w475 w478 w482 w490 w497 w517 w519 w523 w536] -> w235
      tunnel: w234 -> [w248 w297 w399 w404 w413 w417 w418 _ _ w444 w456 w468 w475 w478 w482 w490 w497 w517 w519 w523 w536]
      tunnel: w233 -> [w246 _ _ _ _ _ _ _ _ _ _ _ _ _ _ _ _ _ _ _ _]
      event Timeout {
        n145 = event-data() -> ()  [unwired: 1 in, 1 out]
        n146 = local read "Mode"() -> (w251:T5)
        n147 = case shown="\"Custom\", Default" "Dashboard Tab" {
          tunnel: w254 -> [_ _ w270 _ _]
          tunnel: "TestMode/Automatic/" ("Name Pattern") -> [_ _ w269 _ _]
          tunnel: T23 [{"Operation"=enum."Clear", "Color Box"=14013909}, {"Operation"=enum."Clear", "Color Box"=14013909}, {"Operation"=enum."Clear", "Color Box"=14013909}, {"Operation"=enum."Clear", "Color Box"=14013909}, {"Operation"=enum."Update", "Color Box"=14013909}, {"Operation"=enum."Update", "Color Box"=16777215}, {"Operation"=enum."Clear", "Color Box"=14013909}, {"Operation"=enum."Clear", "Color Box"=14013909}, {"Operation"=enum."Clear", "Color Box"=14013909}] -> [_ _ w262 _ w290]
          tunnel: w251 -> [_ _ w261 _ w289]
          tunnel: u32[] [15790320, 15790320, 15790320, 15790320, 16777215, 16777215, 15790320, 15790320, 15790320] -> [_ _ _ _ w295]
          tunnel: w249 -> [_ _ _ _ w283]
          tunnel: w246 -> [_ w256 _ _ _]
          frame "Custom", Default {
          }
          frame "Basic" {
            n148 = call <vilib>:"WPI_DashboardUpdateNames.vi"("Controls on Tab"=w256) -> ()  [unwired: 11 in]
          }
          frame "Test" {
            w268 = -2 ("Active Item:Row Number")
            n149 = Index Array(array=w262, index=w261) -> (element=w263:T26)
            n150 = Unbundle(w263) -> ("Operation"=w264:enum16{"Update", "Clear"}, "Color Box"=w265:u32)
            n151 = call <vilib>:"NT Read String.vi"("Name"="TestMode/TestName") -> ("String"=w259:string)  [unwired: 9 in, 1 out]
            n152 = call <vilib>:"NT Read and Format Entries as Tree.vi"("Operation"=w264, "Name Pattern"=w269, "Tree Refnum"=w270) -> ()  [unwired: 7 in, 2 out]
            n153 = case shown="\"\"" w259 {
              tunnel: "TestMode/TestProgress" ("Name") -> [w272 _]
              tunnel: "TestMode/TestProgressText" ("Name") -> [w271 _]
              frame Default {
                n154 = call <vilib>:"NT Read Number.vi"("Name"=w272) -> ("Numeric"=w273:dbl)  [unwired: 9 in, 1 out]
                n155 = call <vilib>:"NT Read String.vi"("Name"=w271) -> ("String"=w274:string)  [unwired: 9 in, 1 out]
                n156 = Bundle("Numeric"=w273, "String"=w274) -> (→"Progress":cluster{"Numeric":dbl, "String":string})  [unwired: 1 in]
              }
              frame "" {
                n157 = property on="Progress" class="Clust (strict)"("Visible"=FALSE) -> ()  [unwired: 2 in, 2 out]
                n158 = local write "Test Name"(u16 0) -> ()
              }
            }
            n159 = property on="Test Tree" class="Tree (strict)"("Active Item Row Number"=w268, "ActiveColNum"=w268, "CellBG"=w265, "Active Item Row Number"=-1 ("Active Item:Row Number"), "CellBG"=u32 5789784 ("Color Box")) -> ()  [unwired: 2 in, 2 out]
          }
          frame "Variables" {
            w280 = string[] ["CameraPublisher", "Usage", "DB"]  # Items to initially close
            n160 = First Call?() -> (First Call?: T/F=w281:bool)
            n161 = control-ref of="Tree"() -> (w282:refnum<vi>)
            n162 = Select(t=w280, s=w281, f=string[] []) -> (s? t:f=w278:string[])
            n163 = call <vilib>:"NT Read and Format Entries as Tree.vi"("Tags to  Close"=w278, "Tree Refnum"=w282) -> ()  [unwired: 8 in, 2 out]
          }
          frame "Commands" {
            w291 = u32 5789784 ("Color Box")
            w292 = T27 {"Row"=-1, "Column"=-2} ("Active Cell:Active Cell")
            w294 = T27 {"Row"=-2, "Column"=-2} ("Active Cell:Active Cell")
            n164 = Index Array(array=w295, index=w289) -> (element=w293:u32)
            n165 = Index Array(array=w290, index=w289) -> (element=w288:T26)
            n166 = Unbundle(w288) -> ("Operation"=w287:enum16{"Update", "Clear"})  [unwired: 1 out]
            n167 = local read "Command Selection"() -> (w286:i32)
            n168 = property on="Command Selection" class="MCListbox (strict)"("ActiveCell"=w294, "CellBG"=w293, "ActiveCell"=w292, "CellBG"=w291) -> ()  [unwired: 2 in, 2 out]
            n169 = call <vilib>:"WPI_DashboardUpdate RPC Info.vi"("Operation"=w287) -> ("update"=w285:bool, "commands"=w284:string[][])  [unwired: 9 in]
            n170 = property on="Command Selection" class="MCListbox (strict)"("ItemNames"=w284) -> ()  [unwired: 2 in, 2 out]
            n171 = property on="Command Params" class="Tbl (strict)"("Active Cell"=w294, "Cell BG Color"=w293, "Active Cell"=w292, "Cell BG Color"=w291) -> ()  [unwired: 2 in, 2 out]
            n172 = call <vilib>:"WPI_DashboardUpdate Command Params.vi"("Update"=w285, "NewVal"=w286, "Commands"=w284, "Param Tbl"=w283) -> ()  [unwired: 7 in, 1 out]
          }
        }
        n173 = call <vilib>:"Connextion Info.vi"() -> ("Connected"=→"NT Connection":bool)  [unwired: 10 in, 1 out]
      }
      event "Test Tree": Value Change {
        # "Show appropriate\ncontrols"
        n174 = event-data() -> ("CtlRef"=w300:refnum<vi>, "NewVal"=w298:string)  [unwired: 1 in]
        n175 = call <vilib>:"WPI_UtilitiesGetTreeIOName.vi"("NewVal"=w298, "TreeControl in"=w300) -> ("I/O Name"=w301:string)  [unwired: 9 in]
        n176 = case shown="\"Camera\"" w301 {
          selector: w301 -> [_ w308 _ w330 w339 _]
          tunnel: w298 -> [_ _ w327 w329 _ w346]
          tunnel: cluster{string[]}[] [{["640x480", "320x240", "160x120"]}, {["Auto", "Fixed indoor", "Fixed outdoor 1", "Fixed outdoor 2", "Fixed fluorescent 1", "Fixed fluorescent 2", "Hold current"]}, {["Auto", "Flicker-free 50 Hz", "Flicker-free 60 Hz", "Hold current"]}, {["None", "Prioritize frame rate", "Prioritize image quality"]}, {["Monochrome", "Color"]}] -> [_ _ _ _ _ w345]
          frame Default {
            w303 = FALSE ("Visible")
            w302 = FALSE ("Visible")
            n177 = property on="Motor" class="Clust (strict)"("Visible"=w302) -> ()  [unwired: 2 in, 2 out]
            n178 = property on="Test Ring" class="Ring (strict)"("Visible"=w302) -> ()  [unwired: 2 in, 2 out]
            n179 = property on="Rev/Fwd" class="Clust (strict)"("Visible"=w303) -> ()  [unwired: 2 in, 2 out]
            n180 = property on="On/Off" class="Bool (strict)"("Visible"=w303) -> ()  [unwired: 2 in, 2 out]
            n181 = property on="Test Slider" class="Slide (strict)"("Visible"=w303) -> ()  [unwired: 2 in, 2 out]
          }
          frame "Analog Out", "Motor", "PWM" {
            w309 = FALSE ("Visible")
            n182 = case shown="\"Analog Out\"" w308 {
              tunnel: [1.0 ("Value") -1.0 ("Value") 0.0 ("Value")] -> w307
              tunnel: [255.0 ("Value") 1.0 ("Value") 5.0 ("Value")] -> w306
              tunnel: [128.0 ("Value") 0.0 ("Value") 0.0 ("Value")] -> w305
              tunnel: [64.0 ("Value") 0.5 ("Value") 1.0 ("Value")] -> w304
              frame "PWM" {
              }
              frame "Motor", Default {
              }
              frame "Analog Out" {
              }
            }
            n183 = property on="Motor" class="Clust (strict)"("Visible"=TRUE) -> ()  [unwired: 2 in, 2 out]
            n184 = property on="Value" class="Slide (strict)"("Value"=w305, "Scale.Minimum"=w307, "Scale.Maximum"=w306, "Scale.Increment"=w304) -> ()  [unwired: 2 in, 2 out]
            n185 = property on="On/Off" class="Bool (strict)"("Visible"=w309) -> ()  [unwired: 2 in, 2 out]
            n186 = property on="Test Slider" class="Slide (strict)"("Visible"=w309) -> ()  [unwired: 2 in, 2 out]
            n187 = property on="Test Ring" class="Ring (strict)"("Visible"=w309) -> ()  [unwired: 2 in, 2 out]
            n188 = property on="Rev/Fwd" class="Clust (strict)"("Visible"=w309) -> ()  [unwired: 2 in, 2 out]
          }
          frame "Servo" {
            w325 = FALSE ("Visible")
            n189 = call <vilib>:"NT Read Number.vi"("Name"=w327) -> ("Numeric"=w326:dbl)  [unwired: 9 in, 1 out]
            n190 = property on="Test Slider" class="Slide (strict)"("Visible"=TRUE, "Scale.Maximum"=170.0 ("Scale.Range:Maximum")) -> ()  [unwired: 2 in, 2 out]
            n191 = local write "Test Slider"(w326) -> ()
            n192 = property on="Motor" class="Clust (strict)"("Visible"=w325) -> ()  [unwired: 2 in, 2 out]
            n193 = property on="Rev/Fwd" class="Clust (strict)"("Visible"=w325) -> ()  [unwired: 2 in, 2 out]
            n194 = property on="On/Off" class="Bool (strict)"("Visible"=w325) -> ()  [unwired: 2 in, 2 out]
            n195 = property on="Test Ring" class="Ring (strict)"("Visible"=w325) -> ()  [unwired: 2 in, 2 out]
          }
          frame "Relay", "Solenoid" {
            w328 = FALSE ("Visible")
            n196 = property on="Motor" class="Clust (strict)"("Visible"=w328) -> ()  [unwired: 2 in, 2 out]
            n197 = property on="Test Slider" class="Slide (strict)"("Visible"=w328) -> ()  [unwired: 2 in, 2 out]
            n198 = Search and Replace String(input string=w329, search string="/Value  **", replace string="/Direction") -> (result string=w335:string)  [unwired: 5 in, 3 out]
            n199 = property on="Test Ring" class="Ring (strict)"("Visible"=w328) -> ()  [unwired: 2 in, 2 out]
            n200 = call <vilib>:"NT Read String.vi"("Name"=w335) -> ("String"=w333:string)  [unwired: 9 in, 1 out]
            n201 = Equal?(x="Both directions", y=w333) -> (x = y?=w331:bool)
            n202 = Not(x=w331) -> (.not. x?=w332:bool)
            n203 = property on="Rev/Fwd" class="Clust (strict)"("Visible"=w331) -> ()  [unwired: 2 in, 2 out]
            n204 = property on="On/Off" class="Bool (strict)"("Visible"=w332, "Caption.Text"=w330) -> ()  [unwired: 2 in, 2 out]
          }
          frame "Compressor", "Digital Out" {
            w338 = FALSE ("Visible")
            # "Get direction and finish"
            n205 = property on="Motor" class="Clust (strict)"("Visible"=w338) -> ()  [unwired: 2 in, 2 out]
            n206 = property on="Test Slider" class="Slide (strict)"("Visible"=w338) -> ()  [unwired: 2 in, 2 out]
            n207 = property on="Test Ring" class="Ring (strict)"("Visible"=w338) -> ()  [unwired: 2 in, 2 out]
            n208 = property on="On/Off" class="Bool (strict)"("Visible"=TRUE, "Caption.Text"=w339) -> ()  [unwired: 2 in, 2 out]
            n209 = property on="Rev/Fwd" class="Clust (strict)"("Visible"=FALSE) -> ()  [unwired: 2 in, 2 out]
          }
          frame "Camera" {
            n210 = call <vilib>:"Get Last Path Segment.vi"("String in"=w346) -> ("String out"=w347:string)  [unwired: 10 in]
            n211 = property on="On/Off" class="Bool (strict)"("Visible"=FALSE) -> ()  [unwired: 2 in, 2 out]
            n212 = property on="Motor" class="Clust (strict)"("Visible"=FALSE) -> ()  [unwired: 2 in, 2 out]
            n213 = property on="Rev/Fwd" class="Clust (strict)"("Visible"=FALSE) -> ()  [unwired: 2 in, 2 out]
            n214 = case shown="\"White Balance  **\"" w347 {
              tunnel: w346 -> [w353 w362 w371 w380 w389 _ w395]
              tunnel: w345 -> [w351 w359 w368 w377 w386 _ _]
              frame "Size  **" {
                n215 = Index Array(array=w351) -> (element=w350:cluster{string[]})  [unwired: 1 in]
                n216 = call <vilib>:"NT Read String.vi"("Name"=w353) -> ("String"=w352:string)  [unwired: 9 in, 1 out]
                n217 = Unbundle(w350) -> (w348:string[])
                n218 = Match First String(2:w348, 3:w352) -> (0:w349:i32)  [unwired: 1 out]
                n219 = property on="Test Ring" class="Ring (strict)"("Value"=w349, "Strings []"=w348) -> ()  [unwired: 2 in, 2 out]
                n220 = property on="Test Ring" class="Ring (strict)"("Visible"=TRUE) -> ()  [unwired: 2 in, 2 out]
                n221 = property on="Test Slider" class="Slide (strict)"("Visible"=FALSE) -> ()  [unwired: 2 in, 2 out]
              }
              frame "White Balance  **" {
                n222 = Index Array(array=w359, index=1) -> (element=w360:cluster{string[]})
                n223 = call <vilib>:"NT Read String.vi"("Name"=w362) -> ("String"=w361:string)  [unwired: 9 in, 1 out]
                n224 = Unbundle(w360) -> (w357:string[])
                n225 = Match First String(2:w357, 3:w361) -> (0:w356:i32)  [unwired: 1 out]
                n226 = property on="Test Ring" class="Ring (strict)"("Value"=w356, "Strings []"=w357) -> ()  [unwired: 2 in, 2 out]
                n227 = property on="Test Ring" class="Ring (strict)"("Visible"=TRUE) -> ()  [unwired: 2 in, 2 out]
                n228 = property on="Test Slider" class="Slide (strict)"("Visible"=FALSE) -> ()  [unwired: 2 in, 2 out]
              }
              frame "Exposure  **" {
                n229 = Index Array(array=w368, index=2) -> (element=w369:cluster{string[]})
                n230 = call <vilib>:"NT Read String.vi"("Name"=w371) -> ("String"=w370:string)  [unwired: 9 in, 1 out]
                n231 = Unbundle(w369) -> (w365:string[])
                n232 = Match First String(2:w365, 3:w370) -> (0:w366:i32)  [unwired: 1 out]
                n233 = property on="Test Ring" class="Ring (strict)"("Value"=w366, "Strings []"=w365) -> ()  [unwired: 2 in, 2 out]
                n234 = property on="Test Ring" class="Ring (strict)"("Visible"=TRUE) -> ()  [unwired: 2 in, 2 out]
                n235 = property on="Test Slider" class="Slide (strict)"("Visible"=FALSE) -> ()  [unwired: 2 in, 2 out]
              }
              frame "Exposure Priority  **" {
                n236 = Index Array(array=w377, index=3) -> (element=w378:cluster{string[]})
                n237 = call <vilib>:"NT Read String.vi"("Name"=w380) -> ("String"=w379:string)  [unwired: 9 in, 1 out]
                n238 = Unbundle(w378) -> (w374:string[])
                n239 = Match First String(2:w374, 3:w379) -> (0:w375:i32)  [unwired: 1 out]
                n240 = property on="Test Ring" class="Ring (strict)"("Value"=w375, "Strings []"=w374) -> ()  [unwired: 2 in, 2 out]
                n241 = property on="Test Ring" class="Ring (strict)"("Visible"=TRUE) -> ()  [unwired: 2 in, 2 out]
                n242 = property on="Test Slider" class="Slide (strict)"("Visible"=FALSE) -> ()  [unwired: 2 in, 2 out]
              }
              frame "Color Enable  **" {
                n243 = Index Array(array=w386, index=4) -> (element=w387:cluster{string[]})
                n244 = call <vilib>:"NT Read String.vi"("Name"=w389) -> ("String"=w388:string)  [unwired: 9 in, 1 out]
                n245 = Unbundle(w387) -> (w383:string[])
                n246 = Match First String(2:w383, 3:w388) -> (0:w384:i32)  [unwired: 1 out]
                n247 = property on="Test Ring" class="Ring (strict)"("Value"=w384, "Strings []"=w383) -> ()  [unwired: 2 in, 2 out]
                n248 = property on="Test Ring" class="Ring (strict)"("Visible"=TRUE) -> ()  [unwired: 2 in, 2 out]
                n249 = property on="Test Slider" class="Slide (strict)"("Visible"=FALSE) -> ()  [unwired: 2 in, 2 out]
              }
              frame Default {
                n250 = property on="Test Ring" class="Ring (strict)"("Visible"=FALSE) -> ()  [unwired: 2 in, 2 out]
                n251 = property on="Test Slider" class="Slide (strict)"("Visible"=FALSE) -> ()  [unwired: 2 in, 2 out]
              }
              frame "Brightness  **", "Color Level  **", "Compression  **", "FPS  **", "Sharpness  **" {
                n252 = call <vilib>:"NT Read Number.vi"("Name"=w395) -> ("Numeric"=w394:dbl)  [unwired: 9 in, 1 out]
                n253 = local write "Test Slider"(w394) -> ()
                n254 = property on="Test Slider" class="Slide (strict)"("Visible"=TRUE, "Scale.Maximum"=100.0 ("Scale.Range:Maximum")) -> ()  [unwired: 2 in, 2 out]
                n255 = property on="Test Ring" class="Ring (strict)"("Visible"=FALSE) -> ()  [unwired: 2 in, 2 out]
              }
            }
          }
        }
        n256 = property on="Progress" class="Clust (strict)"("Visible"=FALSE) -> ()  [unwired: 2 in, 2 out]
      }
      event "Test Name": Mouse Enter {
        # "Populate the ring with the list of tests"
        n257 = event-data() -> ()  [unwired: 1 in, 1 out]
        n258 = call <vilib>:"NT Read String Array.vi"("Name"="TestMode/TestList") -> ("String Array"=w403:string[])  [unwired: 9 in, 1 out]
        n259 = Build Array (concatenate)("Select the test to run...", w403) -> (w402:string[])
        n260 = property on="Test Name" class="Ring (strict)"("Strings []"=w402) -> ()  [unwired: 2 in, 2 out]
      }
      event "Test Name": Value Change {
        w405 = FALSE ("Visible")
        # "Tell the robot the test name to run"
        n261 = event-data() -> ("NewVal"=w409:u16)  [unwired: 1 in]
        n262 = property on="Test Name" class="Ring (strict)"() -> ("Strings []"=w410:string[])  [unwired: 2 in, 2 out]
        n263 = local write "Progress"(T7 {"Test Progress"=0, "Test Progress Text"=""} ("Progress")) -> ()
        n264 = Index Array(array=w410, index=w409) -> (element=w408:string)
        n265 = call <vilib>:"NT Write String.vi"("String"=w408, "Name"="TestMode/TestName") -> ()  [unwired: 9 in, 1 out]
        n266 = property on="Progress" class="Clust (strict)"("Visible"=TRUE) -> ()  [unwired: 2 in, 2 out]
        n267 = property on="Motor" class="Clust (strict)"("Visible"=w405) -> ()  [unwired: 2 in, 2 out]
        n268 = property on="Test Slider" class="Slide (strict)"("Visible"=w405) -> ()  [unwired: 2 in, 2 out]
        n269 = property on="On/Off" class="Bool (strict)"("Visible"=w405) -> ()  [unwired: 2 in, 2 out]
        n270 = property on="Rev/Fwd" class="Clust (strict)"("Visible"=w405) -> ()  [unwired: 2 in, 2 out]
        n271 = property on="Test Ring" class="Ring (strict)"("Visible"=w405) -> ()  [unwired: 2 in, 2 out]
      }
      event "Select Auto": Mouse Enter {
        # "Populate the combo box with the list of autonomous options"
        n272 = event-data() -> ()  [unwired: 1 in, 1 out]
        n273 = call <vilib>:"NT Read String Array.vi"("Name"="Auto List") -> ("String Array"=w412:string[])  [unwired: 9 in, 1 out]
        n274 = property on="Select Auto" class="CmbBox"("Strings[]"=w412) -> ()  [unwired: 2 in, 2 out]
      }
      event "Select Auto": Value Change {
        # "User modified the Auto Selection. Write to NT variable so robot knows."
        n275 = event-data() -> ("NewVal"=w415:string)  [unwired: 1 in]
        n276 = call <vilib>:"NT Write String.vi"("String"=w415, "Name"="Auto Selector") -> ()  [unwired: 9 in, 1 out]
      }
      event "Command Selection": Value Change {
        # "Get the params and show in table"
        n277 = event-data() -> ("NewVal"=w421:i32)  [unwired: 1 in]
        n278 = property on="Command Selection" class="MCListbox (strict)"() -> ("ItemNames"=w419:string[][])  [unwired: 2 in, 2 out]
        n279 = call <vilib>:"WPI_DashboardUpdate Command Params.vi"("NewVal"=w421, "Commands"=w419, "Param Tbl"=w420) -> ()  [unwired: 8 in, 1 out]
      }
      event "Execute Command": Value Change {
        # "Started one, Unique ID holds\nresponse"
        n280 = event-data() -> ()  [unwired: 1 in, 1 out]
        n281 = property on="Command Selection" class="MCListbox (strict)"() -> ("ItemNames"=w432:string[][])  [unwired: 2 in, 2 out]
        n282 = Index Array(array=w432, index (row)="Command Selection", index (col)=0) -> (element=w430:string)
        n283 = call <vilib>:"Invoke Commands.vi"("Command Params"="Command Params", "Function Name"=w430) -> ("Params"=w426:u8, "Started"=w425:bool)  [unwired: 7 in, 1 out]
        n284 = Array Subset(array="Command Params", length (row)=w426) -> (w427:string[][])  [unwired: 3 in]
        n285 = Select(t="Executing" ("Cmd Status"), s=w425, f="" ("Cmd Status")) -> (s? t:f=→"Cmd Status":string)
      }
      event "Command Selection": Double Click {
        n286 = event-data() -> ("Row"=w440:i32)  [unwired: 1 in]
        n287 = property on="Command Selection" class="MCListbox (strict)"() -> ("ItemNames"=w443:string[][])  [unwired: 2 in, 2 out]
        n288 = local read "Command Params"() -> (w439:string[][])
        n289 = Index Array(array=w443, index (row)=w440, index (col)=0) -> (element=w441:string)
        n290 = call <vilib>:"Invoke Commands.vi"("Command Params"=w439, "Function Name"=w441) -> ("Params"=w438:u8, "Started"=w433:bool)  [unwired: 7 in, 1 out]
        n291 = Array Subset(array=w439, length (row)=w438) -> (w437:string[][])  [unwired: 3 in]
        n292 = Select(t="Executing" ("Cmd Status"), s=w433, f="" ("Cmd Status")) -> (s? t:f=w434:string)
        n293 = local write "Cmd Status"(w434) -> ()
      }
      event "CheckList": Double Click {
        # "Shift clears all"
        # "Update symbols on the listbox"
        n294 = event-data() -> ("PlatMods.Shift"=w445:bool, "Row"=w447:i32)  [unwired: 1 in]
        n295 = case shown="True" w445 {
          tunnel: w447 -> [w451 _]
          tunnel: 1 -> [w450 _]
          frame False {
            n296 = property on="CheckList" class="LstBox (strict)"() -> ("Item Symbols"=w449:i32[])  [unwired: 2 in, 2 out]
            n297 = Replace Array Subset(array=w449, new element=w450, index=w451) -> (w448:i32[])
            n298 = property on="CheckList" class="LstBox (strict)"("Item Symbols"=w448) -> ()  [unwired: 2 in, 2 out]
          }
          frame True {
            w452 = 0 ("Top Row")
            n299 = property on="CheckList" class="LstBox (strict)"() -> ("Number of Rows"=w454:u32)  [unwired: 2 in, 2 out]
            n300 = Initialize Array(0, w454) -> (w453:i32[])
            n301 = property on="CheckList" class="LstBox (strict)"("Top Row"=w452, "Value"=w452, "Item Symbols"=w453) -> ()  [unwired: 2 in, 2 out]
          }
        }
      }
      event "CheckList": Key Down {
        # "Update symbols on the listbox\nLeft and right keys check and uncheck"
        n302 = event-data() -> ("VKey"=w458:T24)  [unwired: 1 in]
        n303 = case shown="\"Left\", \"Right\"" w458 {
          selector: w458 -> [w463 _]
          tunnel: eventvkey."Left" ("VKey") -> [w461 _]
          frame "Left", "Right" {
            n304 = Equal?(x=w461, y=w463) -> (x = y?=w462:bool)
            n305 = Select(t=0, s=w462, f=1) -> (s? t:f=w464:i32)
            n306 = property on="CheckList" class="LstBox (strict)"() -> ("Item Symbols"=w467:i32[])  [unwired: 2 in, 2 out]
            n307 = Replace Array Subset(array=w467, new element=w464, index="CheckList") -> (w466:i32[])
            n308 = property on="CheckList" class="LstBox (strict)"("Item Symbols"=w466) -> ()  [unwired: 2 in, 2 out]
          }
          frame Default {
          }
        }
      }
      event "Motor.Enable": Value Change {
        # "When the test mode otor enable helper is set, update that\ntree row item's value"
        n309 = event-data() -> ("NewVal"=w473:bool)  [unwired: 1 in]
        n310 = Unbundle("Motor") -> ("Value"=w472:dbl)  [unwired: 1 out]
        n311 = Select(t=w472, s=w473, f=0.0) -> (s? t:f=w470:dbl)
        n312 = call <vilib>:"NT Write Number.vi"("Numeric"=w470, "Name"=w469) -> ()  [unwired: 9 in, 1 out]
      }
      event "Test Slider": Value Change {
        # "When the test mode slider helper is set, update that\ntree row item's value"
        n313 = event-data() -> ("NewVal"=w476:dbl)  [unwired: 1 in]
        n314 = call <vilib>:"NT Write Number.vi"("Numeric"=w476, "Name"=w477) -> ()  [unwired: 9 in, 1 out]
      }
      event "On/Off": Value Change {
        # "When the test mode on/off helper value is set, update that\ntree row item's value"
        n315 = event-data() -> ("NewVal"=w481:bool)  [unwired: 1 in]
        n316 = Boolean To (0,1)(Boolean=w481) -> (0, 1=w480:i16)
        n317 = call <vilib>:"NT Write Number.vi"("Numeric"=w480, "Name"=w479) -> ()  [unwired: 9 in, 1 out]
      }
      event "Rev/Fwd": Value Change {
        # "When the test mode helper value for relays is set, update that\ntree row item's value"
        n318 = event-data() -> ("NewVal.Forward"=w489:bool, "NewVal.Reverse"=w488:bool)  [unwired: 1 in]
        n319 = Boolean To (0,1)(Boolean=w489) -> (0, 1=w485:i16)
        n320 = Boolean To (0,1)(Boolean=w488) -> (0, 1=w487:i16)
        n321 = Negate(x=w487) -> (-x=w486:i16)
        n322 = Add(x=w485, y=w486) -> (x+y=w484:i16)
        n323 = call <vilib>:"NT Write Number.vi"("Numeric"=w484, "Name"=w483) -> ()  [unwired: 9 in, 1 out]
      }
      event "Test Ring": Value Change {
        # "When a test mode helper value is selected from the ring,\nset the tree item's variable to the string value"
        n324 = event-data() -> ("NewVal"=w493:u16)  [unwired: 1 in]
        n325 = property on="Test Ring" class="Ring (strict)"() -> ("Strings []"=w494:string[])  [unwired: 2 in, 2 out]
        n326 = Index Array(array=w494, index=w493) -> (element=w492:string)
        n327 = call <vilib>:"NT Write String.vi"("String"=w492, "Name"=w491) -> ()  [unwired: 9 in, 1 out]
      }
      event "Rec Mode": Value Change {
        # "Update globals for recording mode and path to read log from.\nClear when logging and let NetworkTables set path for vision to\nuse."
        n328 = event-data() -> ("NewVal"=w505:enum32{"Stop", "Record", "Playback"})  [unwired: 1 in]
        n329 = global write "WPI_DashboardLogging Global.vi" "Logging Filename"(path "") -> ()
        n330 = global write "WPI_DashboardLogging Global.vi" "Recording"(w505) -> ()
        n331 = case shown="\"Playback\"" w505 {
          tunnel: w504 -> [_ w507 w516]
          tunnel: [_ _ w515] -> w502
          tunnel: [_ _ w514] -> _
          tunnel: w500 -> [_ _ w512]
          tunnel: cluster{i32, i32} {-250, 170} -> [_ _ w511]
          tunnel: [_ _ T25 {"Image Size"=TRUE, "Image Type"=TRUE, "Pixel Value"=TRUE, "ROI Information"=TRUE, "Zoom Factor"=FALSE} ("Image Information Shown:All Elements")] -> w495
          tunnel: [_ _ TRUE ("Zoom Factor")] -> w496
          tunnel: w498 -> [_ _ w508]
          frame Default {
          }
          frame "Stop", "Record" {
            # "Place Window too"
            n332 = invoke class="VI" method="FP.Close"(reference=w507) -> (reference out=w506:refnum<vi>)  [unwired: 2 in, 2 out]
            n333 = invoke class="VI" method="Abort VI"(reference=w506) -> ()  [unwired: 2 in, 3 out]
          }
          frame "Playback" {
            n334 = call "Open Playback Panel.vi"("Offset"=w511, "DB VI Ref"=w512, "Playback in"=w516) -> ("Playback out"=w513:refnum<vi>)  [unwired: 8 in]
            n335 = register-events(w513, w508) -> (reference out=w515:refnum<event-registration>, error out=w514:errorcluster)  [unwired: 2 in]
          }
        }
        n336 = property on="Camera Image Right" class="ImageControl"("Image Information Shown"=w495, "Image Information Visible"=w496) -> ()  [unwired: 2 in, 2 out]
        n337 = property on="Camera Image" class="ImageControl"("Image Information Shown"=w495, "Image Information Visible"=w496) -> ()  [unwired: 2 in, 2 out]
        n338 = call <vilib>:"WPI_DashboardNT Log FieldName Cache.vi"("Operation"=enum16{"Lookup/Add", "Index", "Clear"}."Clear") -> ()  [unwired: 8 in, 3 out]
      }
      event Panel Close {
        w518 = enum32{"Stop", "Record", "Playback"}."Stop" ("Rec Mode")
        # "Playback window has been closed, abort"
        n339 = event-data() -> ()  [unwired: 1 in, 4 out]
        n340 = local write "Rec Mode"(w518) -> ()
        n341 = global write "WPI_DashboardLogging Global.vi" "Recording"(w518) -> ()
      }
      event Panel Close {
        # "Abort playback window and ourself"
        n342 = event-data() -> ()  [unwired: 1 in, 4 out]
        n343 = invoke class="VI" method="FP.Close"(reference=w522) -> (reference out=w521:refnum<vi>)  [unwired: 2 in, 2 out]
        n344 = invoke class="VI" method="Abort VI"(reference=w521) -> (error out=w520:errorcluster)  [unwired: 2 in, 2 out]
        n345 = invoke class="VI" method="Abort VI"(error in=w520) -> ()  [unwired: 2 in, 3 out]
      }
      event User Event {
        n346 = event-data() -> ("IDs"=w529:cluster{"RPC field ID":u16, "Unique ID":u16}, "String"=w528:string)  [unwired: 1 in]
        n347 = Bundle("IDs"=w529, "String"=w528) -> (w527:T10)  [unwired: 1 in]
        n348 = call <vilib>:"Retrieve RPC Response.vi"("RPC Response"=w527) -> ("Output"=w525:string[][])  [unwired: 10 in]
        n349 = Build Array (concatenate)(w523, w525) -> (w524:string[][])
        n350 = local write "Command Params"(w524) -> ()
        n351 = local write "Cmd Status"("" ("Cmd Status")) -> ()
      }
      event "Tree": Double Click {
        n352 = event-data() -> ("PlatMods"=w535:T28, "Tag"=w532:string)  [unwired: 1 in]
        n353 = Unbundle(w535) -> ("Shift"=w534:bool)  [unwired: 4 out]
        n354 = String Subset(string=w532, length (rest)=1 ("length (rest)")) -> (substring=w531:string)  [unwired: 1 in]
        n355 = Not(x=w534) -> (.not. x?=w533:bool)
        n356 = case shown="\"/\"" w531 {
          tunnel: w532 -> [_ w538]
          tunnel: w533 -> [_ w537]
          frame Default {
          }
          frame "/" {
            n357 = call <vilib>:"NT Update Persistence.vi"("Persistence"=w537, "Name"=w538) -> ()  [unwired: 9 in, 1 out]
          }
        }
      }
    }
  }
  n358 = while {
    tunnel: w65 -> [w540]
    i -> [w543]
    stop <- FALSE stop-if-true
    n359 = Wait (ms)(milliseconds to wait=u32 100) -> ()  [unwired: 1 out]
    n360 = case shown="\"Playback\"" "Rec Mode" {
      tunnel: w543 -> [_ _ w558]
      tunnel: [u32 2829099 ("Base Color") u32 11141120 ("Target Color") w547] -> w539
      frame "Stop", Default {
        # "Reset the color, extra updates don't cost much"
      }
      frame "Record" {
      }
      frame "Playback" {
        # "Playback"
        n361 = Quotient & Remainder(x=w558, y=u32 50 ("milliseconds to wait")) -> (x-y*floor(x/y)=w554:u32)  [unwired: 1 out]
        n362 = Divide(x=w554, y=u32 50 ("milliseconds to wait")) -> (x/y=w551:dbl)
        n363 = Multiply(x=6.283185307179586, y=w551) -> (x*y=w556:dbl)
        n364 = Sine(x=w556) -> (sin(x)=w555:dbl)
        n365 = Absolute Value(x=w555) -> (abs(x)=w548:dbl)
        n366 = call "Interpolate RGB Color.vi"("Proportion"=w548, "Target Color"=u32 30976, "Base Color"=u32 2829099) -> ("Result Color"=w547:u32)  [unwired: 8 in]
      }
    }
    n367 = property class="Pane"(reference=w540, "PaneColor"=w539) -> ()  [unwired: 1 in, 2 out]
  }
  n368 = local write "Dashboard Tab"(T3."Drive" ("Dashboard Tab")) -> ()
  n369 = property on="On/Off" class="Bool (strict)"("Visible"=w36) -> ()  [unwired: 2 in, 2 out]
  n370 = property on="Motor" class="Clust (strict)"("Visible"=w36) -> ()  [unwired: 2 in, 2 out]
  n371 = property on="Progress" class="Clust (strict)"("Visible"=w36) -> ()  [unwired: 2 in, 2 out]
  n372 = property on="Test Ring" class="Ring (strict)"("Visible"=w36) -> ()  [unwired: 2 in, 2 out]
  n373 = property on="Rev/Fwd" class="Clust (strict)"("Visible"=w36) -> ()  [unwired: 2 in, 2 out]
  n374 = while {
    tunnel: u16 1741 ("timeout ms (25000)") -> [w560]
    stop <- FALSE stop-if-true
    n375 = TCP Create Listener(10:w560) -> (0:w559:errorcluster, 3:w561:refnum<k5>)  [unwired: 4 in, 1 out]
    n376 = case shown="No Error" w559 {
      selector: w559 -> [w563 _]
      tunnel: w561 -> [w564 _]
      frame No Error {
        n377 = while {
          tunnel: w564 -> [w567]
          tunnel: w563 -> [w566]
          stop <- FALSE stop-if-true
          n378 = TCP Wait On Listener(8:w566, 11:w567) -> (0:w568:errorcluster, 4:w569:refnum<k5>)  [unwired: 2 in, 3 out]
          n379 = local write "TCP"(w569) -> ()
          n380 = case shown="No Error" w568 {
            frame No Error {
            }
            frame Error {
              n381 = Wait (ms)(milliseconds to wait=u32 1000) -> ()  [unwired: 1 out]
            }
          }
        }
      }
      frame Error {
        n382 = Wait (ms)(milliseconds to wait=u32 1000) -> ()  [unwired: 1 out]
      }
    }
  }
  n383 = local write "Command Selection"(u16 0 ("milliseconds to wait")) -> ()
  n384 = local write "Command Params"(string[][] [] ("Command Params")) -> ()
  n385 = global write "WPI_DashboardLogging Global.vi" "Recording"(w59) -> ()
  n386 = local write "Rec Mode"(w59) -> ()
  n387 = call <vilib>:"NT Write String.vi"("String"="Select Auto", "Name"="Auto Selector") -> ()  [unwired: 9 in, 1 out]
